vi "PCO_GetSensorSignalStatus.vi"(0 "ph":u64, 11 "error in (no error)":errorcluster {"code" format="%x"}) -> (2 "Sensor_Busy":bool, 3 "Sensor_Idle":bool, 4 "ph out":u64, 6 "ErrorMessage":i32 format="%x", 8 "dwImageCount":u32, 13 "Sensor_exposing":bool, 14 "Sensor_readout":bool, 15 "error out":errorcluster {"code" format="%x"})   [LabVIEW 2020, in "SDK.lvlib" / "SpecialCommandsEdge.lvlib"]
doc: "<b>Description:</b>\nThis function returns the current action state of the camera sensor.\nThe delay between the software delivered status and the current status may be several milliseconds due to response and processing times caused by the interface and / or the operating system. For exact synchronization to external events, hardware signals must be used.\n\n<b>Supported camera type:</b>\npco.edge\n\n<b>Descriptor dependency:</b>\nNone"
uses:
  SpecialCommandsEdge.lvlib
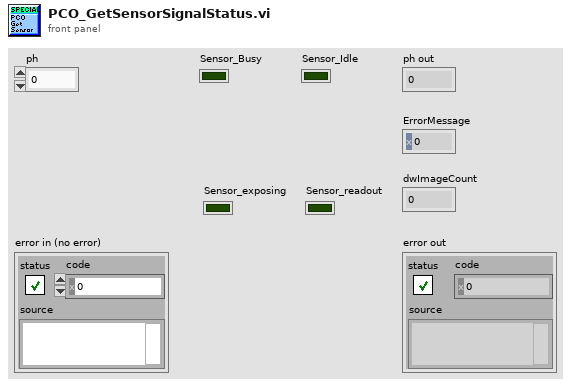
[diagram p1: front panel]
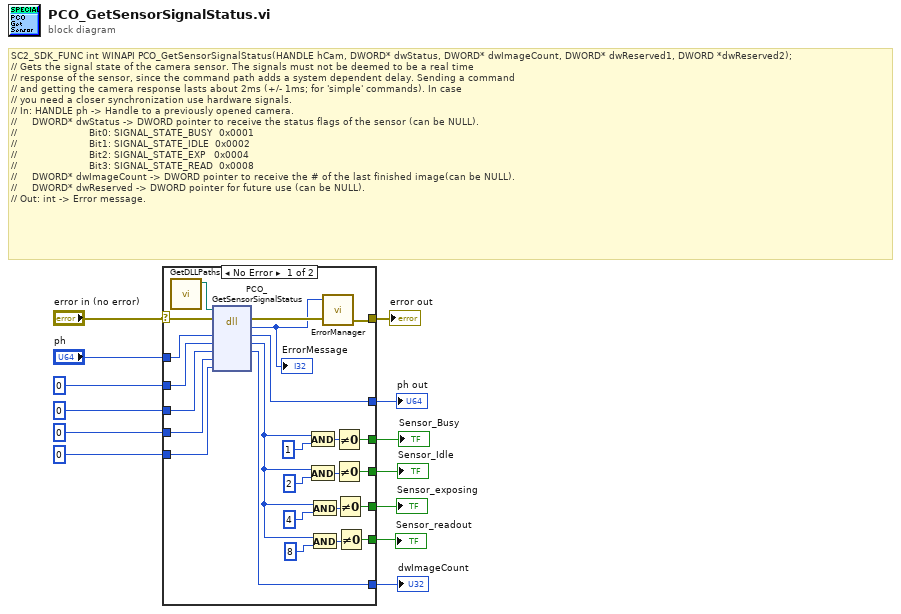
[diagram p0: block diagram]
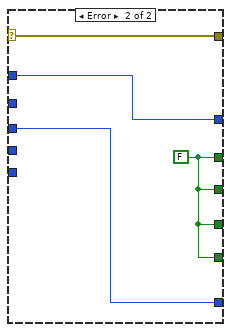
[diagram p2: hidden frame]
diagram:
  # "SC2_SDK_FUNC int WINAPI PCO_GetSensorSignalStatus(HANDLE hCam, DWORD* dwStatus, DWORD* dwImageCount, DWORD* dwReserved1, DWORD *dwReserved2);\n// Gets the signal state of the camera sensor. The signals must not be deemed to be a real time\n// response of the sensor, since the command path adds a system dependent delay. Sending a command\n// and getting the camera response lasts about 2ms (+/- 1ms; for 'simple' commands). In case\n// you need a closer synchronization use hardware signals.\n// In: HANDLE ph -> Handle to a previously opened camera.\n//     DWORD* dwStatus -> DWORD pointer to receive the status flags of the sensor (can be NULL).\n//                        Bit0: SIGNAL_STATE_BUSY  0x0001\n//                        Bit1: SIGNAL_STATE_IDLE  0x0002\n//                        Bit2: SIGNAL_STATE_EXP   0x0004\n//                        Bit3: SIGNAL_STATE_READ  0x0008\n//     DWORD* dwImageCount -> DWORD pointer to receive the # of the last finished image(can be NULL).\n//     DWORD* dwReserved -> DWORD pointer for future use (can be NULL).\n// Out: int -> Error message."
  n1 = case shown="No Error" "error in (no error)" {
    selector: "error in (no error)" -> [w18 w42]
    tunnel: "ph" -> [w38 w41]
    tunnel: [w37 w41] -> w12
    tunnel: u32 0 ("dwImageCount") -> [w36 w39]
    tunnel: [w35 w39] -> w10
    tunnel: u32 0 ("dwReserved1") -> [w34 _]
    tunnel: u32 0 ("dwReserved2") -> [w33 _]
    tunnel: [w16 w42] -> w7
    tunnel: u32 0 ("dwImageCount") -> [w32 _]
    tunnel: [w22 w40] -> w5
    tunnel: [w21 w40] -> w4
    tunnel: [w20 w40] -> w3
    tunnel: [w19 w40] -> w2
    frame No Error {
      n2 = call "GetDLLPaths.vi"() -> ("SC2_Cam_Path"=w14:path)  [unwired: 9 in, 2 out]
      n3 = dll-call lib="?" fn="PCO_GetSensorSignalStatus"(path in=w14, error in=w18, "ph"=w38, "dwStatus"=w32, "dwImageCount"=w36, "dwReserved1"=w34, "dwReserved2"=w33) -> (error out=w17:errorcluster, "return type"=w15:i32, "ph"=w37:u64, "dwStatus"=w28:u32, "dwImageCount"=w35:u32)  [unwired: 3 in, 1 out]
      "ErrorMessage" <- w15
      n4 = And(x=w28, y=u32 1) -> (x .and. y?=w26:u32)
      n5 = And(x=w28, y=u32 2) -> (x .and. y?=w25:u32)
      n6 = And(x=w28, y=u32 4) -> (x .and. y?=w24:u32)
      n7 = And(x=w28, y=u32 8) -> (x .and. y?=w23:u32)
      n8 = call "ErrorManager.vi"("error in (no error)"=w17, "error code"=w15) -> ("error out"=w16:errorcluster)  [unwired: 3 in]
      n9 = Not Equal To 0?(x=w26) -> (x != 0?=w19:bool)
      n10 = Not Equal To 0?(x=w25) -> (x != 0?=w20:bool)
      n11 = Not Equal To 0?(x=w24) -> (x != 0?=w21:bool)
      n12 = Not Equal To 0?(x=w23) -> (x != 0?=w22:bool)
    }
    frame Error {
      w40 = FALSE
    }
  }
  "ph out" <- w12
  "dwImageCount" <- w10
  "error out" <- w7
  "Sensor_Busy" <- w2
  "Sensor_Idle" <- w3
  "Sensor_exposing" <- w4
  "Sensor_readout" <- w5
